vi "Write Label.vi"(8 "error in (no error)":errorcluster, 10 "Label":string, 11 "GenericController in":refnum<class "GenericController.lvclass">) -> (0 "error out":errorcluster, 3 "GenericController out":refnum<class "GenericController.lvclass">)   [LabVIEW 2020, in "GenericController.lvlib" / "GenericController.lvclass"]
uses:
  GenericController.lvclass
  GenericController.lvclass/GenericController.ctl
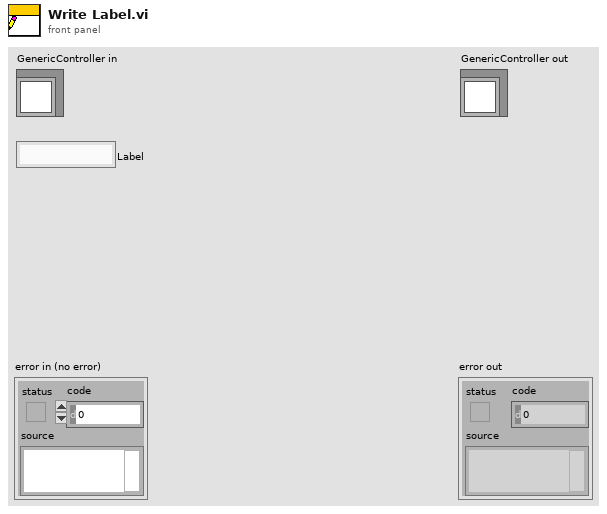
[diagram p1: front panel]
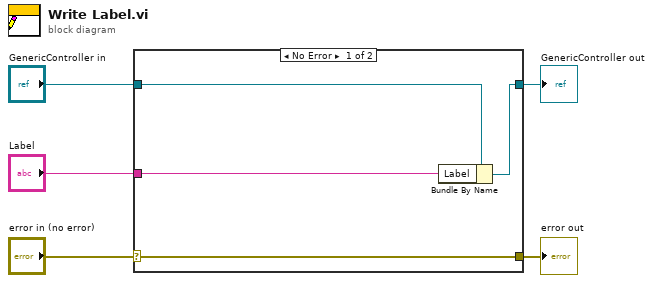
[diagram p0: block diagram]
diagram:
  n1 = case shown="No Error" "error in (no error)" {
    selector: "error in (no error)" -> [w9 w10]
    tunnel: [w9 w10] -> w4
    tunnel: [w7 w11] -> w2
    tunnel: "GenericController in" -> [w8 w11]
    tunnel: "Label" -> [w6 _]
    frame No Error {
      n2 = Bundle By Name(cluster=w8, "Label"=w6) -> (w7:refnum<class "GenericController.lvclass">)
    }
    frame Error {
    }
  }
  "error out" <- w4
  "GenericController out" <- w2
